vi "Configure Data Clock.vi"(6 "External Reference Frequency (13 MHz)":dbl=13000000.0, 7 "External Data Clock (0: Normal)":u16(ring) items=["Normal", "Symbol"], 8 "error in (no error)":errorcluster, 9 "Reference Source (0: Internal)":u16(ring) items=["Internal", "External"], 10 "Data Clock Source (0: Internal)":u16(ring) items=["Internal", "External"], 11 "VISA resource name":refnum<visa-resource-name>) -> (0 "error out":errorcluster, 3 "VISA resource name out":refnum<visa-resource-name>)   [LabVIEW 2014, in "Agilent PSG MXG Series.lvlib"]
doc: "Configures the data clock and the bit-clock.\n\n<B>Notes:</B>\n(1) This VI is valid only in E8267C, E8267D, N5172B, N5182B.\n\n(2) For E8267C, this VI is valid only when the instrument installs <B>Option 002</B> (Internal baseband generator) or <B>Option 602</B> (Digital bus baseband generator).\n\n(3) For E8267D, this VI is valid only when the instrument installs <B>Option 601</B> or <B>Option 602</B> (Internal baseband generator).\n\n(4) For N5172B and N5182B, this VI is valid only when the instrument installs <B>Option 431</B>."
uses:
  Agilent PSG MXG Series.lvlib
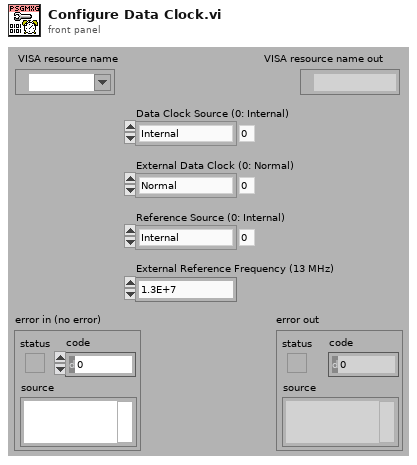
[diagram p1: front panel]
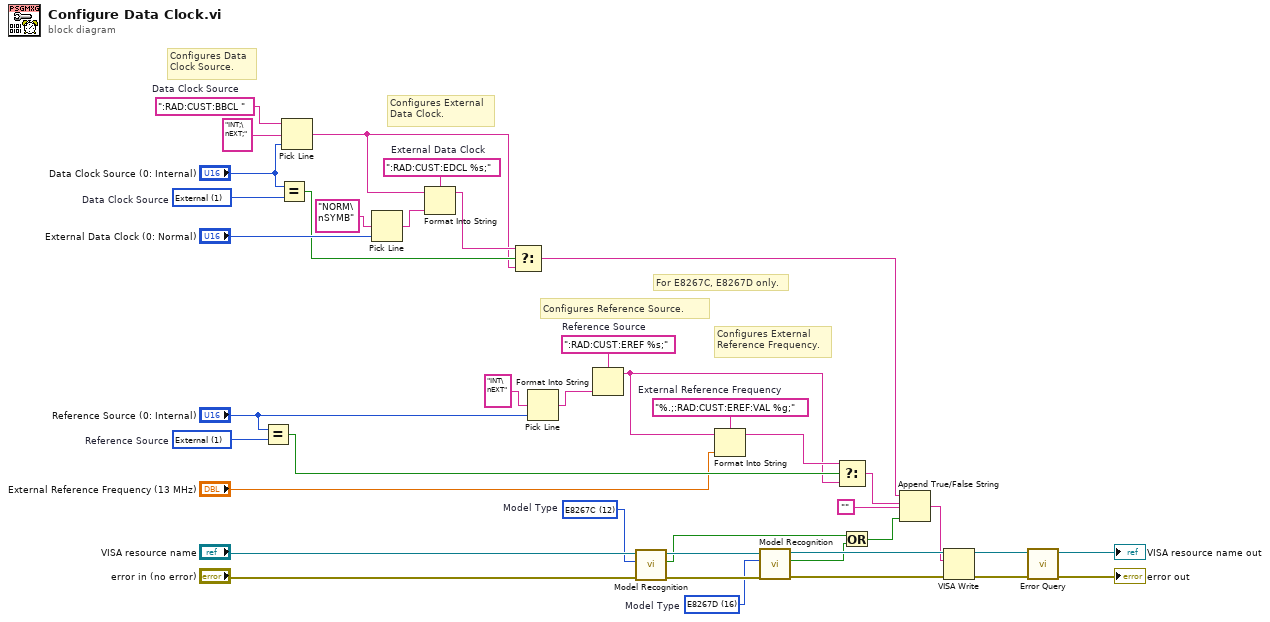
[diagram p0: block diagram]
diagram:
  w5 = u16 16 items=["N5181A"=0, "N5182A"=1, "N5183A"=2, "N5161A"=3, "N5162A"=4, "E8241A"=5, "E8244A"=6, "E8251A"=7, "E8254A"=8, "E8247C"=10, "E8257C"=11, "E8267C"=12, "E8257D"=15, "E8267D"=16, "N5171B"=17, "N5172B"=18, "N5181B"=19, "N5182B"=20]  # Model Type
  w6 = u16 12 items=["N5181A"=0, "N5182A"=1, "N5183A"=2, "N5161A"=3, "N5162A"=4, "E8241A"=5, "E8244A"=6, "E8251A"=7, "E8254A"=8, "E8247C"=10, "E8257C"=11, "E8267C"=12, "E8257D"=15, "E8267D"=16, "N5171B"=17, "N5172B"=18, "N5181B"=19, "N5182B"=20]  # Model Type
  w25 = u16 1 items=["Internal", "External"]  # Data Clock Source
  w20 = ":RAD:CUST:EREF %s;"  # Reference Source
  w32 = u16 1 items=["Internal", "External"]  # Reference Source
  w34 = "%.;:RAD:CUST:EREF:VAL %g;"  # External Reference Frequency
  w38 = ":RAD:CUST:EDCL %s;"  # External Data Clock
  w40 = ":RAD:CUST:BBCL "  # Data Clock Source
  # "For E8267C, E8267D only."
  # "Configures External\nReference Frequency."
  # "Configures Reference Source."
  # "Configures External\nData Clock."
  # "Configures Data\nClock Source."
  n1 = Equal?(x="Reference Source (0: Internal)", y=w32) -> (x = y?=w31:bool)
  n2 = Equal?(x="Data Clock Source (0: Internal)", y=w25) -> (x = y?=w24:bool)
  n3 = Pick Line(string ("")=w40, multi-line string="INT;\nEXT;", line index="Data Clock Source (0: Internal)") -> (output string=w22:string)
  n4 = Pick Line(multi-line string="NORM\nSYMB", line index="External Data Clock (0: Normal)") -> (output string=w21:string)  [unwired: 1 out]
  n5 = Format Into String(format string=w38, initial string=w22, w21) -> (resulting string=w23:string)  [unwired: 1 in, 1 out]
  n6 = Select(t=w23, s=w24, f=w22) -> (s? t:f=w10:string)
  n7 = Pick Line(multi-line string="INT\nEXT", line index="Reference Source (0: Internal)") -> (output string=w19:string)  [unwired: 1 out]
  n8 = Format Into String(format string=w20, w19) -> (resulting string=w18:string)  [unwired: 2 in, 1 out]
  n9 = call "Model Recognition.vi"("error in (no error)"="error in (no error)", "Model Type (0: N5181A)"=w6, "VISA resource name"="VISA resource name") -> ("error out"=w13:errorcluster, "Is Model Correct"=w1:bool, "VISA resource name out"=w4:refnum<visa-resource-name>)  [unwired: 6 out]
  n10 = Format Into String(format string=w34, initial string=w18, "External Reference Frequency (13 MHz)") -> (resulting string=w30:string)  [unwired: 1 in, 1 out]
  n11 = call "Model Recognition.vi"("error in (no error)"=w13, "Model Type (0: N5181A)"=w5, "VISA resource name"=w4) -> ("error out"=w11:errorcluster, "Is Model Correct"=w2:bool, "VISA resource name out"=w12:refnum<visa-resource-name>)  [unwired: 6 out]
  n12 = Select(t=w30, s=w31, f=w18) -> (s? t:f=w8:string)
  n13 = Or(x=w1, y=w2) -> (x .or. y?=w3:bool)
  n14 = Append True/False String(1:w3, 2:"", 3:w8, 4:w10) -> (0:w9:string)
  n15 = VISA Write(VISA resource name=w12, write buffer=w9, error in (no error)=w11) -> (VISA resource name out=w28:refnum<visa-resource-name>, error out=w27:errorcluster)  [unwired: 1 out]
  n16 = call "Error Query.vi"("error in (no error)"=w27, "VISA resource name"=w28) -> ("error out"=→"error out":errorcluster, "VISA resource name out"=→"VISA resource name out":refnum<visa-resource-name>)  [unwired: 8 out]
